vi "Join Game.vi"(8 "error in (no error)":errorcluster, 10 "Your name":string, 11 "CS++GoBangClient in":refnum<class "CS++GoBangClient.lvclass">) -> (0 "error out":errorcluster, 3 "CS++GoBangClient out":refnum<class "CS++GoBangClient.lvclass">)   [LabVIEW 2014, in "GoBang.lvlib" / "CS++GoBangClient.lvclass"]
uses:
  CS++GoBangClient.lvclass
  CS++GoBangClient.lvclass/CS++GoBangClient.ctl
  GoBang.lvlib
  CSPP_Core/Classes/CS++ProcessVariables/PVConnection/PVConnection.lvclass
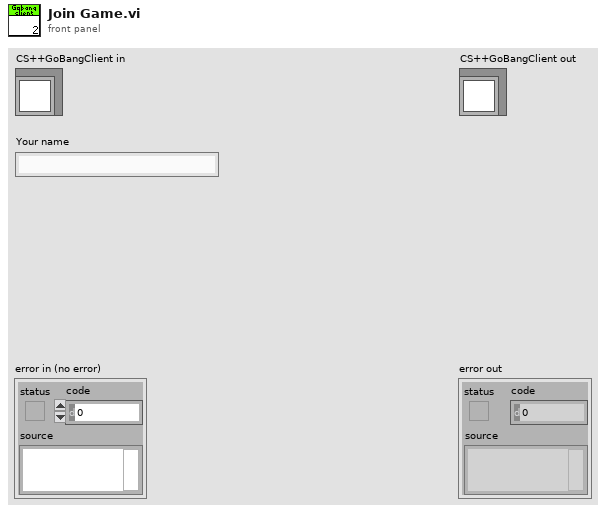
[diagram p1: front panel]
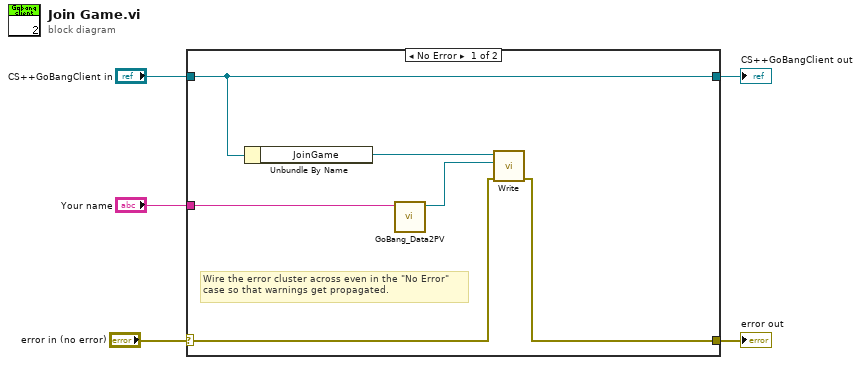
[diagram p0: block diagram]
diagram:
  n1 = case shown="No Error" "error in (no error)" {
    selector: "error in (no error)" -> [w7 w13]
    tunnel: [w6 w13] -> w4
    tunnel: [w10 w12] -> w2
    tunnel: "CS++GoBangClient in" -> [w10 w12]
    tunnel: "Your name" -> [w8 _]
    frame No Error {
      # "Wire the error cluster across even in the \"No Error\"\ncase so that warnings get propagated."
      n2 = Unbundle By Name(w10) -> ("JoinGame"=w9:refnum<class "PVConnection.lvclass">)
      n3 = call "GoBang_Data2PV.vi"("Data in"=w8) -> ("PV out"=w11:refnum<class "PV.lvclass">)  [unwired: 10 in]
      n4 = call "Write.vi"("error in (no error)"=w7, "PV"=w11, "PVConnection in"=w9) -> ("error out"=w6:errorcluster)  [unwired: 7 in, 1 out]
    }
    frame Error {
    }
  }
  "error out" <- w4
  "CS++GoBangClient out" <- w2
